vi "configuration_rm_imu.vi"() -> (3 "configuration_rm_imu":T1={"chunk"=4096, "mode"=1, "_reserved_0"=0, "_reserved_1"=0, "_reserved_2"=0, "_reserved_3"=0, "_reserved_4"=0, "_reserved_5"=0, "_reserved_6"=0})   [LabVIEW 2023]
panel:
  in  "configuration_rm_imu":T1={"chunk"=4096, "mode"=1, "_reserved_0"=0, "_reserved_1"=0, "_reserved_2"=0, "_reserved_3"=0, "_reserved_4"=0, "_reserved_5"=0, "_reserved_6"=0}
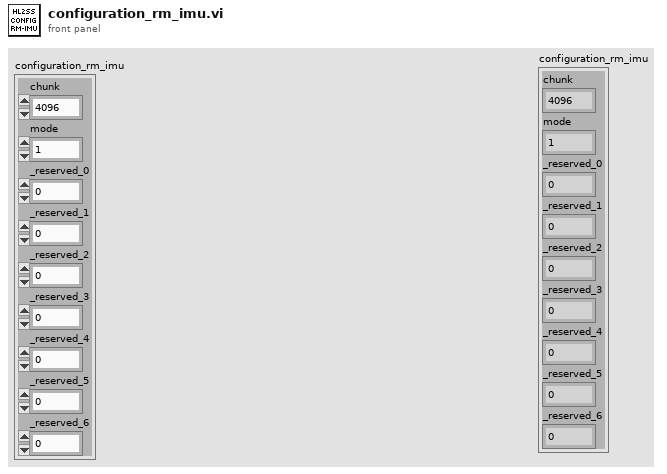
[diagram p1: front panel]
types:
  T1 = cluster{"chunk":u64, "mode":u8, "_reserved_0":u8, "_reserved_1":u8, "_reserved_2":u8, "_reserved_3":u8, "_reserved_4":u8, "_reserved_5":u8, "_reserved_6":u8}
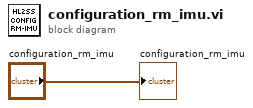
[diagram p0: block diagram]
diagram:
  "configuration_rm_imu" <- "configuration_rm_imu"
